vi "testy.vi"() -> ()   [LabVIEW 2021]
panel:
  out "slave1":dbl
  out "master":dbl
  in  "stop":bool
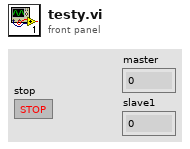
[diagram p1: front panel]
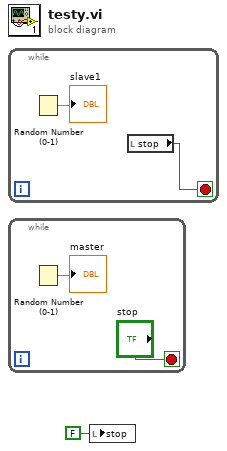
[diagram p0: block diagram]
diagram:
  n1 = while {
    stop <- w2 stop-if-true
    n2 = Random Number (0-1)() -> (number: 0 to 1=→"slave1":dbl)
    n3 = local read "stop"() -> (w2:bool)
  }
  n4 = while {
    stop <- "stop" stop-if-true
    n5 = Random Number (0-1)() -> (number: 0 to 1=→"master":dbl)
  }
  n6 = local write "stop"(FALSE ("stop")) -> ()
